vi "WorkorderHandler_getData(Locked).vi"(0 "reference":T1, 3 "timeout in ms (-1)":i32=-1, 5 "error in (no error)":errorcluster) -> (14 "duplicate reference":T1, 16 "data":T2, 17 "data locked?":bool, 18 "timed out?":bool, 19 "error out":errorcluster)   [LabVIEW 2011]
doc: "Returns the data of the dqGOOP object even if it is locked. The locked data will only be available if the data was locked using getDataToModify(StoreLocked) function."
uses:
  DataStructures/WorkorderHandler_ObjectReference.ctl
  DataStructures/WorkorderHandler_ObjectData.ctl
panel:
  # "Copyright (C) 2004 DataAct Incorporated"
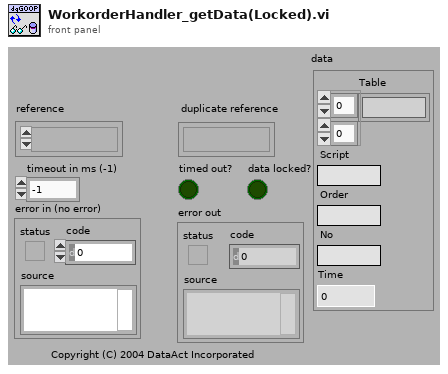
[diagram p1: front panel]
types:
  T1 = typedef "WorkorderHandler_ObjectReference.ctl" = refnum<k1>
  T2 = typedef "WorkorderHandler_ObjectData.ctl" = cluster{"Table":string[][], "Script":string, "Order":string, "No":string, "Time":dbl}
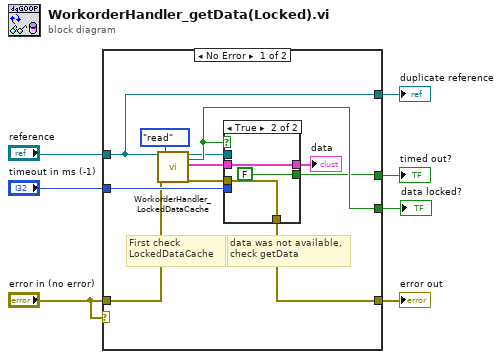
[diagram p0: block diagram]
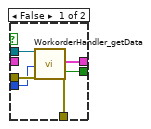
[diagram p2: hidden frame]
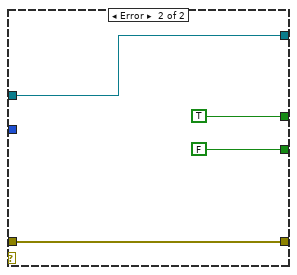
[diagram p3: hidden frame]
diagram:
  n1 = case shown="No Error" "error in (no error)" {
    tunnel: [w12 w29] -> w7
    tunnel: [w10 TRUE] -> w2
    tunnel: "reference" -> [w9 w30]
    tunnel: [w9 w30] -> w5
    tunnel: "timeout in ms (-1)" -> [w14 _]
    tunnel: "error in (no error)" -> [w13 w29]
    tunnel: [w11 FALSE] -> w1
    frame No Error {
      # "data was not available,\ncheck getData"
      # "First check\nLockedDataCache"
      n2 = call "WorkorderHandler_LockedDataCache.vi"("reference"=w9, "error in (no error)"=w13, "action (read)"=enum16{"push", "read", "pop"}."read" ("action")) -> ("reference dup"=w8:T1, "found"=w11:bool, "data out"=w15:T2, "error out"=w17:errorcluster)  [unwired: 1 in, 12 out]
      n3 = case shown="True" w11 {
        tunnel: w17 -> [w24 w26]
        tunnel: [w23 w27] -> w16
        tunnel: w15 -> [_ w27]
        tunnel: w14 -> [w22 _]
        tunnel: [w21 w26] -> w12
        tunnel: [w20 FALSE] -> w10
        tunnel: w8 -> [w19 _]
        frame False {
          n4 = call "WorkorderHandler_getData.vi"("reference"=w19, "timeout in ms (-1)"=w22, "error in (no error)"=w24) -> ("data"=w23:T2, "timed out?"=w20:bool, "error out"=w21:errorcluster)  [unwired: 14 out]
        }
        frame True {
        }
      }
      "data" <- w16
    }
    frame Error {
    }
  }
  "error out" <- w7
  "duplicate reference" <- w5
  "timed out?" <- w2
  "data locked?" <- w1
